vi "Add Monitoring Tags.vi"(8 "error in (no error)":errorcluster, 9 "subscription ID":u32, 10 "OPC UA client refnum":T1, 11 "OPC UA in":refnum<class "OPC UA.lvclass">) -> (0 "error out":errorcluster, 3 "OPC UAout":refnum<class "OPC UA.lvclass">)   [LabVIEW 2021, in "OPC UA.lvclass"]
uses:
  OPC UA.lvclass
  <vilib>/OPCUA/controls/OPC UA Client Refnum.ctl
  OPC UA.lvclass/OPC UA.ctl
  <vilib>/OPCUA/NI OPC UA Client.lvlib
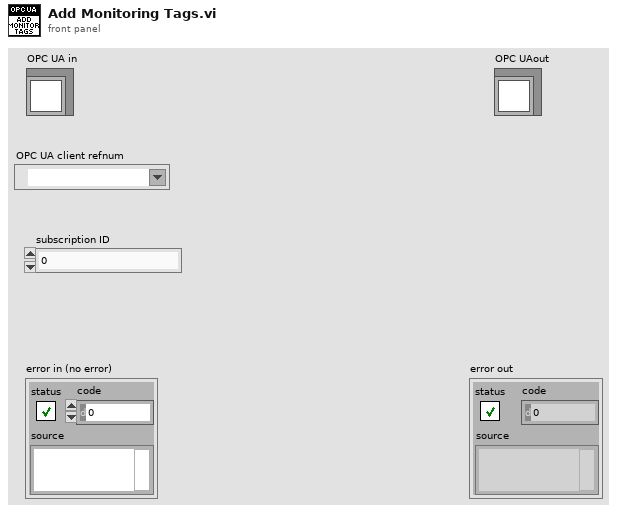
[diagram p1: front panel]
types:
  T1 = typedef "OPC UA Client Refnum.ctl" = refnum<k21>
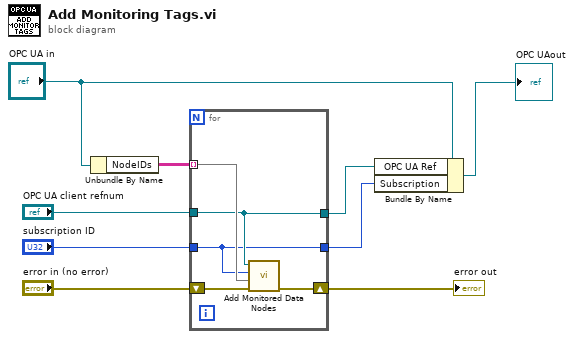
[diagram p0: block diagram]
diagram:
  n1 = Unbundle By Name("OPC UA in") -> ("NodeIDs"=w5:string[][])
  n2 = for {
    shift-right: [w14] -> w8
    shift-left: "error in (no error)" -> [w13]
    tunnel: w5 -> [w12] mode=indexing
    tunnel: "OPC UA client refnum" -> [w11]
    tunnel: "subscription ID" -> [w10]
    tunnel: [w11] -> w3
    tunnel: [w10] -> w1
    n3 = call <vilib>:"Add Monitored Data Nodes.vi"("error in (no error)"=w13, "node IDs"=w12, "subscription ID in"=w10, "OPC UA client refnum in"=w11) -> ("error out"=w14:errorcluster)  [unwired: 4 in, 3 out]
  }
  "error out" <- w8
  n4 = Bundle By Name(cluster="OPC UA in", "OPC UA Ref"=w3, "Subscription"=w1) -> (→"OPC UAout":refnum<class "OPC UA.lvclass">)
